vi "Holding Register Get Starting Address.vi"(8 "error in (no error)":errorcluster, 11 "Item Ref in":T1 format="%.0x") -> (0 "error out":errorcluster, 2 "Value":u16, 3 "Item Ref out":T1 format="%.0x")   [LabVIEW 2015]
uses:
  <vilib>/NI VeriStand/Custom Device API/Custom Device API.lvlib
  Shared/Constants.vi
  Shared/Modbus Master Shared.lvlib
  <vilib>/NI Veristand/Custom Device API/Get Item Property (U16).vi
  <vilib>/NI Veristand/Custom Device API/Custom Device Item Ref.ctl
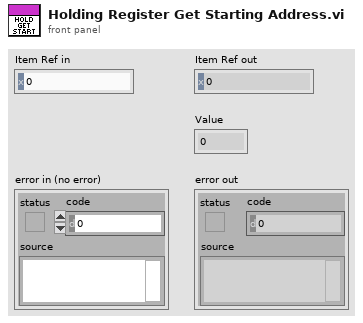
[diagram p1: front panel]
types:
  T1 = typedef "Custom Device API.lvlib/Custom Device Item Ref.ctl" = u64
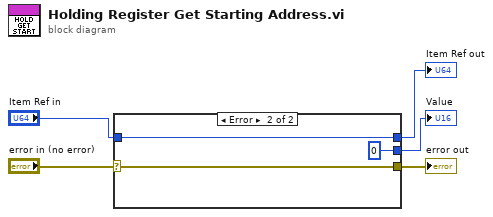
[diagram p0: block diagram]
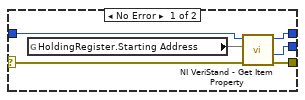
[diagram p2: hidden frame]
diagram:
  n1 = case shown="Error" "error in (no error)" {
    selector: "error in (no error)" -> [w10 w13]
    tunnel: "Item Ref in" -> [w9 w14]
    tunnel: [w8 w13] -> w3
    tunnel: [w7 u16 0 ("Value")] -> w2
    tunnel: [w6 w14] -> w1
    frame No Error {
      n2 = global read "Constants.vi" "HoldingRegister.Starting Address"() -> (w11)
      n3 = call-poly <vilib>:"NI VeriStand - Get Item Property.vi"("error in (no error)"=w10, "Property Name"=w11, "Item Ref in"=w9) -> ("error out"=w8:errorcluster, "Value"=w7:u16, "Item Ref out"=w6:T1)  [unwired: 5 in, 1 out]
    }
    frame Error {
    }
  }
  "error out" <- w3
  "Value" <- w2
  "Item Ref out" <- w1
